vi "AlliGator Color Parameter Map in Original Image.vi"(5 "Color Scale Refnum":refnum<vi>, 7 "Image Color Scale Refnum":refnum<vi>, 8 "Error In":errorcluster, 10 "Destination Image Control Refnum":T1 caption="Source Image Refnum", 11 "AlliGator IV DVR in":refnum<data-value>) -> (0 "Error Out":errorcluster, 1 "# Overlay Pixels":i32, 3 "AlliGator IV DVR out":refnum<data-value>)   [LabVIEW 2021, in "AlliGator Parameter Map.lvlib"]
doc: "Overlays the Decay Fit Parameter Map on the Source Image."
uses:
  AlliGator Parameter Map.lvlib
  Image/Image Control Refnum.ctl
  Internal Variables/AlliGator Internal Variables v2.ctl
  <vilib>/vision/Image Controls.llb/IMAQ Image.ctl
  Internal Variables/AlliGator Gate Image Set.ctl
  Files/AlliGator FLI Dataset Type.ctl
  Files/AlliGator Data Series Type.ctl
  Dual-Channel Datasets/AlliGator Dataset Channel.ctl
  Settings/AlliGator Gate Arithmetic.ctl
  Source Image/AlliGator Displayed Image.ctl
  Image/Named ROI Description.ctl
  Phasor Graph/AlliGator Decay Metadata v3.ctl
  Decay Analysis/Decay Preprocessing/AlliGator Decay Background Subtraction Info.ctl
  Decay Analysis/Decay Preprocessing/AlliGator Baseline Subtraction Method.ctl
  Graphs/XY Graph/XY Graph Plot Shift Parameters.ctl
  Graphs/XY Graph/XY Graph Plot Shift Method.ctl
  Decay Analysis/Decay Preprocessing/AlliGator Decay Extrapolation Parameters.ctl
  Phasor/Calibration Phasor (m, phi).ctl
  Phasor/Phasor Reference Series.ctl
  Phasor/Phasor Calibration Map v2.ctl
  Phasor/Phasor (g, s).ctl
  Phasor Graph/AlliGator Raw Phasor Plot Data v4.ctl
  Phasor/Phasor Standard Deviation Options.ctl
  Phasor Plot/AlliGator Phasor Multi-Harmonic Data.ctl
  Phasor/Phasor Harmonic Data.ctl
  Decay Fit Parameter Map/AlliGator Decay Fit Options & Parameters v2.ctl
  Fits/IRF(X)PSED/Decay Fit Options v2.ctl
  Fits/Decay Convolution/Decay Model.ctl
  Fits/Residual Type.ctl
  Fits/IRF(X)PSED/Fit Weights Type.ctl
  Fits/Non-linear Fitting Method v2.ctl
  Fits/Fit Calculation Method.ctl
  Fits/Non-linear Fitting Algorithm.ctl
  Decay Analysis/Decay Fit/AlliGator Decay Fit Parameter Constraints 2.ctl
  Fits/IRF(X)PSED/Decay Fit Parameters In List.ctl
  Fits/IRF(X)PSED/MLE Baseline Offset Type.ctl
  Decay Analysis/Decay Preprocessing/AlliGator Decay Preprocessing Parameters.ctl
  Fits/IRF(X)PSED/Decay Fit Parameters & Derived Quantities List v2.ctl
  Decay Fit Parameter Map/AlliGator Parameter Maps Data.ctl
  Settings/AlliGator Settings List.ctl
  Globals, Variables, Constants/AlliGator Variables List.ctl
  Palette/Image Palette Information.ctl
  Image/Image Display Palette Type.ctl
  Variant/Variant to Data/Variant to Boolean.vi
  Error/Error.lvlib
  Image/Image.lvlib
  Settings/AlliGator Settings.lvlib
  Variant/Variant to Data/Variant to Data.lvlib
  <vilib>/vision/NI_Vision_Development_Module.lvlib
  Time/Time.lvlib
  Globals, Variables, Constants/AlliGator Globals, Variables & Constants.lvlib
  Palette/Palette.lvlib
  Utilities/Utilities.lvlib
  Phasor/Phasor.lvlib
  Decay Analysis/Decay Preprocessing/AlliGator Decay Preprocessing.lvlib
  Graphs/XY Graph/XY Graph Add-Ons.lvlib
  Phasor Graph/AlliGator Phasor Graph.lvlib
  Files/AlliGator Files.lvlib
  Phasor Plot/AlliGator Phasor Plot.lvlib
  Source Image/AlliGator Source Image.lvlib
  Internal Variables/AlliGator Internal Variables.lvlib
  Fits/Fits.lvlib
  Decay Analysis/Decay Fit/AlliGator Decay Fit.lvlib
  Decay Fit Parameter Map/AlliGator Decay Fit Parameter Map.lvlib
  Dual-Channel Datasets/AlliGator Dual-Channel Datasets.lvlib
panel:
  out "Overlay Copy (s)":dbl
  out "Overlay Erase (s)":dbl
  out "Overlay Compute (s)":dbl
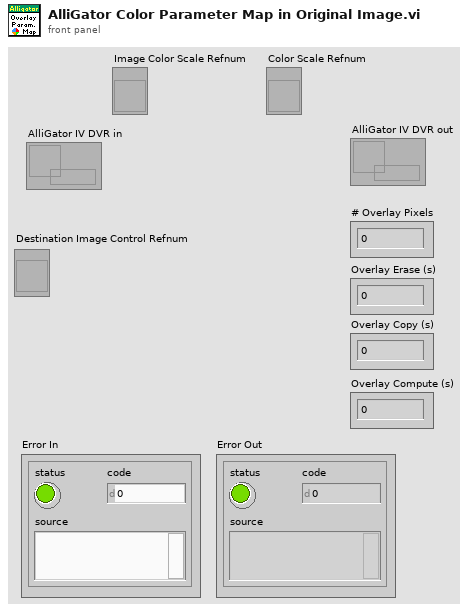
[diagram p1: front panel]
types:
  T1 = typedef "Image.lvlib/Image Control Refnum.ctl" = refnum<vi>
  T2 = typedef "AlliGator Settings.lvlib/AlliGator Settings List.ctl" = enum16{"GUI:Visible Settings Tab", "GUI:Last Run Version", "Source Image:Use Image Histogram for Contrast", "Source Image:Low Count Pixels Rejection Options", "Source Image:High Count Pixels Rejection Options", "Source Image:Use Image Brightness", "Source Image:Blend Overlay with Image Background", "Source Image:Use Fixed ROI Diameter", "Source Image:ROI Diameter", "Source Image:ROI Center Color", "Source Image:Peak Threshold", "Source Image:Intensity Threshold", "Source Image:Image Binning Options", "Source Image:Image Smoothing Options", "Source Image:Image Histogram Active", "Source Image:Invert Binary Mask", "Source Image:Hot Pixel Removal", "Source Image:Overlay Analyzed ROI Center", "Source Image:Auto-Adjust Contrast", "Source Image:Histogram Lower Percentile", "Source Image:Histogram Upper Percentile", "Source Image:Save Source Image", "Source Image:Scale Bar Options", "Source Image:Image Resolution (Pixel Size)", "Source Image:Flatfield Correction", "Source Image:Show Dead Left Columns Correction", "Source Image:Dead Left Columns Correction", "Source Image:Image Pre-Processing Operations Order", "Source Image:Overlay ROI Median", "Source Image:Median Overlay Color", "Data Information:Gate Width", "Data Information:Nanotime Gate Separation", "Data Information:Macrotime Gate Separation", "Data Information:Gate Step", "Data Information:# Gates", "Data Information:Gate Image Exposure", "Data Information:Gate Image Integration", "Data Information:Gates to Skip", "Data Information:Gates to Keep", "Data Information:Define Gates to", "Data Information:Channel Name", "Data Information:Available Channel Names", "Data Information:Channel Arithmetic", "Data Information:Background File Subtraction", "Data Information:Background File", "Data Information:Background Scaling Factor", "Data Information:Background Pile-up Correction", "Data Information:Background Pixel Well Capacity", "Data Information:Laser Period", "Data Information:SYNC Period", "Data Information:Pile-up Correction", "Data Information:Pixel Well Capacity", "Data Information:Dataset Scaling Factor", "Fluorescence Decay_Decay Pre-Processing:Reverse Gates", "Fluorescence Decay_Decay Pre-Processing:Verbose Decay Pre-Processing", "Fluorescence Decay_Decay Pre-Processing:Use Decay Pre-Processing", "Fluorescence Decay_Decay Pre-Processing:Background Subtraction", "Fluorescence Decay_Decay Pre-Processing:Background Definition Range", "Fluorescence Decay_Decay Pre-Processing:Baseline Subtraction Method", "Fluorescence Decay_Decay Pre-Processing:Decay Pre-Processing Operations Order", "Fluorescence Decay_Decay Pre-Processing:Smoothing Parameter", "Fluorescence Decay_Decay Pre-Processing:Shift Decay", "Fluorescence Decay_Decay Pre-Processing:Decay Shift Parameters", "Fluorescence Decay_Decay Pre-Processing:Fold Decay", "Fluorescence Decay_Decay Pre-Processing:# Folds", "Fluorescence Decay_Decay Pre-Processing:1-Normalize Decay", "Fluorescence Decay_Decay Pre-Processing:[0-1]-Normalize Decay", "Fluorescence Decay_Decay Pre-Processing:Smoothen Decay", "Fluorescence Decay_Decay Pre-Processing:Extrapolate Decay", "Fluorescence Decay_Decay Pre-Processing:Use Periodicity", "Fluorescence Decay_Decay Pre-Processing:Use Cursors", "Fluorescence Decay_Decay Pre-Processing:Tail Fraction", "Fluorescence Decay_Decay Pre-Processing:Head Fraction", "Fluorescence Decay_Decay Pre-Processing:Additional Points", "Fluorescence Decay_Decay Pre-Processing:Straighten Decay", "Fluorescence Decay_Decay Pre-Processing:Constant Background", "Fluorescence Decay_Decay Pre-Processing:Pixel-Normalize Decay", "Fluorescence Decay_Advanced Analysis:Extract IRF instead of Decay", "Fluorescence Decay_Advanced Analysis:IRF Extraction Options", "Fluorescence Decay_Advanced Analysis:IRF Optimization Options", "Fluorescence Decay_Advanced Analysis:Square Pulse Options", "Fluorescence Decay_Advanced Analysis:IRF Order", "Fluorescence Decay_Advanced Analysis:IRF Time Constants", "Fluorescence Decay_Advanced Analysis:Wavelet Analysis Options", "Fluorescence Decay_Advanced Analysis:Average Lifetime Options", "Fluorescence Decay_Fit Options:Fit Options", "Fluorescence Decay_Fit Options:Use Legacy Fitting Approach", "Fluorescence Decay_Fit Options:Use Data Information Laser Period", "Fluorescence Decay_Fit Parameters:Displayed Fit Parameters", "Fluorescence Decay_Fit Parameters:Fit Parameter Constraints", "Fluorescence Decay_Fit Parameters:Export Tabulated Results", "Fluorescence Decay_Fit Parameters:MLE Baseline Offset Type", "Fluorescence Decay_Fit Parameters:MLE Baseline Offset", "Fluorescence Decay_Fit Parameters:Guess Parameter Names", "Fluorescence Decay_Fit Parameters:Guess Parameter Values", "Fluorescence Decay_Fit Parameters:Guess Parameters Options", "Fluorescence Decay_Fit Parameters:Optimal Offset Selection Criterion", "Fluorescence Decay_Styles:Show Last Decay Only", "Fluorescence Decay_Styles:Decay Graph Color Array", "Fluorescence Decay:Decay Graph Active", "Fluorescence Decay Statistics:Min Peak Value", "Fluorescence Decay Statistics:Reject Low Decay Peak Pixels", "Fluorescence Decay Statistics:Reject High Decay Peak Pixels", "Fluorescence Decay Statistics:Max Peak Value", "Time Traces:Use File Timestamp", "Time Traces:Time Step", "Time Traces:Use Intensity Correction File", "Time Traces:Intensity Correction File", "Phasor Plot:Phasor Plot Smoothing Options", "Phasor Plot:Phasor Plot Size", "Phasor Plot:Phasor Plot Graphics Options", "Phasor Plot:Cumulative Phasor Plot", "Phasor Plot:Use Phasor Brightness", "Phasor Plot:Blend Overlay with Phasor Background", "Phasor Plot:Save Phasor Plot", "Phasor Plot:Show References", "Phasor Plot:Phasor Ratio Decay Range", "Phasor Plot:Exponential Fading", "Phasor Plot:Phasor Ratio Reference Colors", "Phasor Plot:Reference Radius", "Phasor Plot:Show Color Map Vertices", "Phasor Plot:Phasor Plot Active", "Phasor Plot:Phasor Ratio Color Map Type", "Phasor Plot:Phasor Ratio Color Map", "Phasor Plot:Phasor Ratio Display Range", "Phasor Plot:Selected Image ROI(s)", "Phasor Plot:All Image ROIs", "Phasor Plot:Selected Phasor Plot ROI(s)", "Phasor Plot:All Phasor Plot ROIs", "Phasor Plot:Phasor Ratio Color-Coded Quantity", "Phasor Plot:Store Phasor Harmonics", "Phasor Plot:Draw Reference Segment", "Phasor Plot:User-Defined Quantity", "Phasor Plot:Color Scale High Color", "Phasor Plot:Color Scale Low Color", "Phasor Graph:Phasor Frequency", "Phasor Graph:Phasor Ratio Type", "Phasor Graph:Pixel-level Phasor Computation", "Phasor Graph:Save Phasor Graph", "Phasor Graph:Phasor Graph Active", "Phasor Graph:Phasor SDV Options", "Phasor Calibration:Use Backup Calibration if needed", "Phasor Graph:Define Shortest Lifetime as", "Phasor Calibration:Backup Calibration Type", "Phasor Calibration:Calibration Type", "Phasor Calibration:Calibration Lifetime", "Phasor Calibration:Calibration Map Algorithm", "Single-Exponential Phasor Locus (SEPL):Gate Parameters", "Single-Exponential Phasor Locus (SEPL):User-defined Gate", "Single-Exponential Phasor Locus (SEPL):User-defined IRF", "Single-Exponential Phasor Locus (SEPL):Phasor Parameters", "Single-Exponential Phasor Locus (SEPL):Decay & IRF Parameters", "Single-Exponential Phasor Locus (SEPL):Display Parameters", "Lifetime Analysis:Decay Analysis Parameters", "Lifetime Analysis:Lifetime Map Active", "Plugins:Python Settings", "Miscellaneous:Verbose Mode", "Miscellaneous:Beep after Script", "Miscellaneous:Saved Image File Format", "Miscellaneous:Exported Gate Image Settings", "Miscellaneous:Include Loading in Timing", "Miscellaneous:Verbose Settings Mode", "Miscellaneous:Histogram Options", "Miscellaneous:Beep on Error", "Miscellaneous:# Logical Processors Used", "Miscellaneous:ROI Description Max Characters", "Miscellaneous:Verbose Error Mode", "Miscellaneous:Transparent Mask Color"}
  T3 = typedef "IMAQ Image.ctl" = refnum<image>
  T4 = typedef "AlliGator Globals, Variables & Constants.lvlib/AlliGator Variables List.ctl" = enum16{"---- GUI ----", "GUI:Initialization Status", "GUI:State Indicators Refnum", "GUI:Original AlliGator Menu Items", "GUI:Current Action Loop State", "GUI:Script in progress", "GUI:Playback", "GUI:Loop Playback", "GUI:Search ROI Used", "GUI:Search ROI", "Decay Graph Max Legend Size", "Intensity Graph Max Legend Size", "Decay Statistics Graph Max Legend Size", "Phasor Graph Max Legend Size", "Phasor Ratio Graph Max Legend Size", "Lifetime Graph Max Legend Size", "---- Files ----", "Files:Export Dataset Frames as Individual Files", "Files:Show Batch Export Help Balloons", "Files:Frames in Dataset", "Files:ptu File Frame Start Indices", "Files:Current Frame in Dataset", "Files:Current Frame Timestamp", "Files:Dataset Loaded", "Files:Dataset Metadata", "Files:Dataset Channel", "Files:Dataset Data Description", "Files:Background Dataset Metadata", "Files:Background Dataset Channel", "Files:Background Dataset Data Description", "Files:Background File Subtraction", "Files:Background File Path", "Files:Background File Pile-up Correction", "Files:Background File Pixel Well Capacity", "Files:Background File Scaling Factor", "Files:Current Dataset Load Settings", "Files:Dataset Path", "Files:ICCD-specific Information", "Files:Macrotime Gate Separation", "------ Python Plugins ------", "Python Plugins:Information", "Python Plugins:Python Session", "Python Plugins:Valid Python Session?", "---- Source Image ----", "Source Image:ROIs", "Source Image:Current ROI", "Source Image:ROI Event Refnum", "X_Source Image:Display Range", "X_Source Image:Palette Information", "X_Source Image:Type of Displayed Image", "X_Time Gate Slider", "Source Image:Palette List", "Source Image:Scale", "Source Image:ROI Overlay Color", "Source Image:Overlay to Erase", "Source Image:Is Displayed Image Accumulated", "Source Image:White Light Image Modified", "Source Image:Mask Image Modified", "---- Image Profile Window ----", "Image Profile:Window Event Refnum", "Image Profile:IntensityType", "Image Profile:Intensity Average Type", "Image Profile:Intensity-weighted SDV", "Image Profile:Box Profile Type", "Image Profile:Window Open", "Image Profile:Plotted Fit Parameter", "------ Phasor Graph -------", "Phasor Graph:Show Line", "---- Phasor Plot ---", "Phasor Plot:Parameters Changed", "Phasor Plot:FLI Dataset Modified since last Calculation", "Phasor Harmonics Data", "Selected Phasor Harmonics", "Phasor Harmonic Manager Event Refnum", "Phasor Plot:ROIs", "Phasor Plot:Current ROI", "Phasor Plot:ROI Event Refnum", "Phasor Plot:Image Reference Points", "Phasor Plot:Computed", "Phasor Plot:Palette Information", "Phasor Plot:Palette List", "Phasor Plot:Phasor Ratio Palette Information", "Phasor Plot:Phasor Ratio Palette List", "Phasor Plot:Image Scale", "Phasor Plot:Image Overlay to Erase", "Phasor Plot:Image Elements to Update", "Phasor Plot:Current Calculation Parameters", "Phasor Plot:Current Calibration Options", "Phasor Plot:Reset Cumulated Phasor Plot", "Phasor Plot:Reference 1", "Phasor Plot:Lifetime Reference 1", "Phasor Plot:Reference 1 Frequency", "Phasor Plot:Reference 2", "Phasor Plot:Lifetime Reference 2", "Phasor Plot:Reference 2 Frequency", "---- Decay Analysis ----", "Number of Selected Decays to Fit", "LS Fit Results", "LAR Fit Results", "BS Fit Results", "Last Decay Max - Min", "Best Fit Parameters", "Best Fit Parameter Names", "Actual Size X", "Actual Size Y", "Binning X", "Binning Y", "Actual # Gates", "Dataset Number", "Gates to...", "Gates Skipped", "Gates to keep", "Gate Step", "Gate Separation", "Reversed Gates", "Pile-up Correction", "Pixel Well Capacity", "Background Subtracted", "Background Subtraction Method", "Background Definition Range", "Background File (deprecated)", "Number of Dataset Accumulated", "Array of Accumulated Dataset Paths", "Do Averaged Datasets", "Destination File Path", "Process Plot Target", "Use 1/D as Phasor Frequency", "---- Decay Fit Parameter Map -----", "Decay Fit Parameter Map:Palette Information", "Decay Fit Parameter Map:Palette List", "Decay Fit Parameter Map:X Resolution", "Decay Fit Parameter Map:Y Resolution", "---- Parameter Map ----", "Parameter Map:Palette Information", "Parameter Map:Palette List", "------- Local Decay Window ---------", "Local Decay Graph Window:Event Refnum", "Local Decay Graph Window:Use normalized IRF for convolution", "----- Miscellaneous ----", "Misc:Skippable Dialog Windows Status"}
  T5 = typedef "Palette.lvlib/Image Palette Information.ctl" = cluster{"Palette Name [# Colors,int?,inv?]":string, "Palette Type":T6, "Palette Colors":u32[], "Interpolate?":bool}
  T6 = typedef "Image.lvlib/Image Display Palette Type.ctl" = u32
  T7 = typedef "AlliGator Internal Variables.lvlib/AlliGator Internal Variables v2.ctl" = cluster{"Displayed Image":T3, "White Light Image":T3, "Mask Image":T3, "ROI Mask Image":T3, "Current Dataset Images 1":T8, "Background Dataset Images 1":T8, "Current Dataset Images 2":T8, "Background Dataset Images 2":T8, "Current Dataset Arithmetic Images":T8, "Accumulated Dataset Images 1":T8, "Accumulated Dataset Images 2":T8, "Accumulated Dataset Arithmetic Images":T8, "Phasor Plot Image":T3, "Decay Fit Parameter Map Image":T3, "Parameter Map Image":T3, "Single Data Point Path":path, "White Light Image Path":path, "Mask Image Path":path, "Time-Series Folder":path, "[Time-Series Paths]":path[], "Current Dataset":i32, "Single Dataset Type":T9, "Current Folder":string, "AlliGator Data Series Type":T10, "# Datasets":i32, "Dual-Channel Dataset":bool, "Selected Channel Name":string, "Dataset Channel":T11, "Channel Arithmetic":T12, "Dual-Channel Background Dataset":bool, "Background Channel":T11, "Dual-Channel Accumulated Dataset":bool, "Start Time":dbl, "[Time-Series Timestamps]":dbl[], "[Intensity Corrections]":dbl[], "Time Series Script":bool, "Type of Displayed Image":T13, "Gate Image Slide":u16, "# Gates":i32, "ROIs":T14[], "ROI Decay":cluster{"t Array":dbl[], "I Array":dbl[]}, "Valid Decay":bool, "Decay  Metadata":T16, "Reference Decay Plot Name":string, "Reference Decay":cluster{"t Array":dbl[], "I Array":dbl[]}, "Decay Shift Plot":cluster{"Time Stamps":dbl[], "Decay Shifts":dbl[]}, "[Decays Max Values]":sgl[], "[Decays Min Values]":sgl[], "Calibration Phasor":T22, "Calibration Phasor Series":T23, "Phasor Calibration Map":T24, "Calibration Map MD5 Digest":string, "Last Raw Phasor":T25, "Last Calibrated Phasor":T25, "Last Calibrated Phasor SDV":T25, "Phasor Graph:Phasor Plot":cluster{"g Array":dbl[], "s Array":dbl[]}, "Phasor Graph:Phasor SDV Plot":cluster{"g Array":dbl[], "s Array":dbl[]}, "[Phasor Graph:Raw Phasor Plots]":T26[], "Phasor Plot locked to Ref 1":i32, "[Phasor Plot(s) locked to Ref 1]":i32[], "[Phasor Plot(s) locked to Ref 2]":i32[], "[Pixel Phasors]":T25[], "[[Sum Image]]":dbl[][], "[[CSG Phasors]]":csg[][], "[[Valid Pixel?]]":bool[][], "I/m/phi Dataset":cluster{"I/m/phi Dataset?":bool, "Base Frequency":dbl[unit], "Harmonic Orders":u8[]}, "Multi Phasor Plot Data":T28, "Decay Fit Options & Parameters":T30, "Fit Options: Decay Preprocessing Parameters":T41, "Fit Options: Reference Decay":cluster{"t Array":dbl[], "I Array":dbl[]}, "Is Full Image Parameters Map":bool, "Is Single-Pixels Parameters Map":bool, "NLSF Parameters Map X Resolution":i32, "NLSF Parameters Map Y Resolution":i32, "[Single Decay Fit Parameters]":dbl[], "Fit Model":T32, "[[Multiple Decays Fit Parameters]]":dbl[][], "[[Multiple Decays Fit Parameter SDVs]]":dbl[][], "[[IRFs]]":dbl[][], "IRF Array Time Axis":dbl[], "Decay Array Time Axis":dbl[], "[Decay Fit Parameter Names]":T42[], "[[Phasor Ratios]]":dbl[][], "[[Average Lifetimes]]":dbl[][], "Amplitude Weighted Average Lifetime":bool, "[Decay Sum]":dbl[], "[Map Set Names]":string[], "[Parameter Maps]":T43[], "[[User-defined Quantities]]":dbl[][], "User-defined Quantity":string}
  T8 = typedef "AlliGator Internal Variables.lvlib/AlliGator Gate Image Set.ctl" = cluster{"SGL Image Max":T3, "SGL Image Sum":T3, "SGL Gate Images":T3[], "SGL Image Min":T3}
  T9 = typedef "AlliGator Files.lvlib/AlliGator FLI Dataset Type.ctl" = enum16{"HDF5 FLI Dataset", "Gate Image Folder", ".sdt FLI Dataset (Becker & Hickl)", ".ptu FLI Dataset (PicoQuant)", "SS1 FLI Dataset", "SS2 FLI Dataset", "I/m/phi Dataset", ".bin FLI Dataset (PicoQuant Binned)", ".bin FLI Dataset (Piccolo Binned)", ".mat FLI Dataset"}
  T10 = typedef "AlliGator Files.lvlib/AlliGator Data Series Type.ctl" = enum16{"Not a Supported Series", "Gate Images Folder Series", "SwissSPAD 2 Dataset Series", "B&H FLI Dataset Series", "PicoQuant PTU FLI Dataset Series", "PicoQuant BIN FLI Dataset Series", "Piccolo hist BIN FLI Dataset Series", "HDF5 FLI Dataset Series"}
  T11 = typedef "AlliGator Dual-Channel Datasets.lvlib/AlliGator Dataset Channel.ctl" = enum16{"G2", "INT"}
  T12 = typedef "AlliGator Settings.lvlib/AlliGator Gate Arithmetic.ctl" = enum16{"None", "INT-G2", "G2/INT*<INT>", "(1 - G2/INT)*<INT>"}
  T13 = typedef "AlliGator Source Image.lvlib/AlliGator Displayed Image.ctl" = enum16{"Single Gate", "Sum of All Gates", "Max of All Gates", "Min of All Gates", "-", "White Ligth Image", "Mask Image"}
  T14 = typedef "Image.lvlib/Named ROI Description.ctl" = cluster{"ROI Descriptor":T15, "ROI Name":string, "Overlay Color":u32}
  T15 = typedef "ROI Descriptor" = cluster{"Global Rectangle":i32[], "Contours":cluster{"ID":enum32{"External", "Internal"}, "Type":u32, "Coordinates":i32[]}[]}
  T16 = typedef "AlliGator Phasor Graph.lvlib/AlliGator Decay Metadata v3.ctl" = cluster{"ROI Descriptor":T15, "ROI Center":cluster{"X":i32, "Y":i32}, "Decay Background Subtraction Info":T17, "Decay Reverted":bool, "Decay Smoothened":bool, "Decay Straightened":bool, "Fitted Tau (Decay Straightening)":dbl, "Decay Shift Parameters":T19, "Decay Shifted":bool, "Decay Extrapolated":bool, "Decay Extrapolation Parameters":T21, "Decay Normalized":bool, "Fold Decay":bool, "# Folds":u32}
  T17 = typedef "AlliGator Decay Preprocessing.lvlib/AlliGator Decay Background Subtraction Info.ctl" = cluster{"Laser Period":dbl[unit], "Gate Duration":dbl[unit], "Baseline Subtraction Method":T18, "Background Definition Range":cluster{"Min Gate":dbl[unit], "Max Gate":dbl[unit]}, "Total Intensity w/o Bkgd Subtraction":dbl, "Bkgd-subtracted Intensity (exp)":dbl, "# Data Points":i32, "Background/Gate":dbl, "Fitted Lifetime":dbl[unit], "Bkgd-subtracted Intensity (theo)":dbl}
  T18 = typedef "AlliGator Decay Preprocessing.lvlib/AlliGator Baseline Subtraction Method.ctl" = enum16{"Mean", "Min", "Square Gated Single-Exponential", "File", "Constant"}
  T19 = typedef "XY Graph Add-Ons.lvlib/XY Graph Plot Shift Parameters.ctl" = cluster{"Type":T20, "Shift":dbl[unit], "Threshold":dbl, "Rotate":bool}
  T20 = typedef "XY Graph Add-Ons.lvlib/XY Graph Plot Shift Method.ctl" = enum16{"Default", "CFD", "Threshold", "Cross-Correlation"}
  T21 = typedef "AlliGator Decay Preprocessing.lvlib/AlliGator Decay Extrapolation Parameters.ctl" = cluster{"Additional Points":u32, "Head Fraction":dbl, "Fitted Tau":dbl, "Use Periodicity":bool, "Use Cursors":bool, "Tail Fraction":dbl}
  T22 = typedef "Phasor.lvlib/Calibration Phasor (m, phi).ctl" = cluster{"m":dbl, "phi":dbl, "Phasor Frequency":dbl[unit], "Reference Lifetime":dbl[unit]}
  T23 = typedef "Phasor.lvlib/Phasor Reference Series.ctl" = cluster{"m Array":dbl[], "phi Array":dbl[], "Phasor Frequency":dbl[unit], "Calibration Lifetime":dbl[unit]}
  T24 = typedef "Phasor.lvlib/Phasor Calibration Map v2.ctl" = cluster{"Phasor Frequency":dbl[unit], "Calibration Lifetime":dbl[unit], "ROI Centers":cluster{"X":i32, "Y":i32}[], "ROI Descriptors":T15[], "Map Resolution X":i32, "Map Resolution Y":i32, "z Array":cdb[]}
  T25 = typedef "Phasor.lvlib/Phasor (g, s).ctl" = cluster{"g":dbl, "s":dbl}
  T26 = typedef "AlliGator Phasor Graph.lvlib/AlliGator Raw Phasor Plot Data v4.ctl" = cluster{"Phasor Plot Name":string, "Raw Phasor Plot":T25[], "Phasor Frequency":dbl[unit], "[Decay Metadata]":T16[], "Raw Phasor Plot SDV":T25[], "Phasor SDV Options":T27, "[Calibration Phasor]":T22[]}
  T27 = typedef "Phasor.lvlib/Phasor Standard Deviation Options.ctl" = cluster{"Compute Estimated SDV":bool, "# Replicas":u32, "Use Estimated Average Phasor":bool}
  T28 = typedef "AlliGator Phasor Plot.lvlib/AlliGator Phasor Multi-Harmonic Data.ctl" = cluster{"Base Frequency":dbl[unit], "# Harmonics":u8, "Harmonic Orders":u8[], "Phasor Plot Settings Checksum":u64, "Phasor Harmonic Data Array":T29[]}
  T29 = typedef "Phasor.lvlib/Phasor Harmonic Data.ctl" = cluster{"Phasor Harmonic Name":string, "Phasor Plot Settings Checksum":u64, "Phasor Frequency":dbl[unit], "Base Frequency":dbl[unit], "Harmonic Order":u8, "Phasor Plot Parameters":string, "Phasor Array [[CSG]]":csg[][], "Dataset File Path":path}
  T30 = typedef "AlliGator Decay Fit Parameter Map.lvlib/AlliGator Decay Fit Options & Parameters v2.ctl" = cluster{"SYNC Period":dbl[unit], "Fit Options":T31, "Fit Parameter Constraints":T38[], "MLE Baseline Offset":dbl, "MLE Baseline Offset Type":T40}
  T31 = typedef "Fits.lvlib/Decay Fit Options v2.ctl" = cluster{"Show Fit Residuals":bool, "Fit Model":T32, "Residual Type":T33, "Max Decay Percentile":dbl, "Min Decay Percentile":dbl, "Show Full Decay":bool, "Weights":T34, "Fitting Method":T35, "Compute Parameter Uncertainties":bool, "Periodic Boundaries":bool, "Model Calculation":T36, "Period":dbl[unit], "Termination Criteria":cluster{"Max Iterations":i32, "Max Function Calls":i32, "Max Time":dbl[unit], "Function Tolerance":dbl, "Parameter Tolerance":dbl, "Gradient Tolerance":dbl, "Min Lambda":dbl, "Max Lambda":dbl, "Initial Tick Count":u32}, "Offset Resolution":dbl[unit], "Use Local IRF":bool, "Fitting Algorithm":T37}
  T32 = typedef "Fits.lvlib/Decay Model.ctl" = enum16{"1-Exponential", "2-Exponentials"}
  T33 = typedef "Fits.lvlib/Residual Type.ctl" = enum16{"Standard", "Normalized", "Reduced"}
  T34 = typedef "Fits.lvlib/Fit Weights Type.ctl" = enum16{"Unweighted", "1/Variance", "Best of All"}
  T35 = typedef "Fits.lvlib/Non-linear Fitting Method v2.ctl" = enum16{"Least Square", "Least Absolute Residual", "Bisquare", "MLE", "-", "Best of All"}
  T36 = typedef "Fits.lvlib/Fit Calculation Method.ctl" = enum16{"Simulation", "Convolution", "Integration"}
  T37 = typedef "Fits.lvlib/Non-linear Fitting Algorithm.ctl" = enum16{"Levenberg-Marquardt", "Trust-Region Dogleg"}
  T38 = typedef "AlliGator Decay Fit.lvlib/AlliGator Decay Fit Parameter Constraints 2.ctl" = cluster{"Fit Parameter":T39, "Min Value":dbl, "Max Value":dbl, "Global":bool, "Used":bool}
  T39 = typedef "Fits.lvlib/Decay Fit Parameters In List.ctl" = enum16{"Offset", "Baseline", "A_1", "tau_1", "A_2", "tau_2"}
  T40 = typedef "Fits.lvlib/MLE Baseline Offset Type.ctl" = enum32{"Absolute", "Percentage"}
  T41 = typedef "AlliGator Decay Preprocessing.lvlib/AlliGator Decay Preprocessing Parameters.ctl" = cluster{"Background Subtraction":bool, "Straighten Decay":bool, "Reverse Gates":bool, "1-Normalized Decay":bool, "Smoothen Decay":bool, "Smoothing Parameter":dbl, "Shift Decay":bool, "Decay Shift Parameters":T19, "Extrapolate Decay":bool, "Additional Points":u32, "Head Fraction":dbl, "Pixel-Normalize Decay":bool, "Use Periodicity":bool, "Use Cursors":bool, "Tail Fraction":dbl, "Use Decay Pre-Processing":bool, "Fold Decay":bool, "# Folds":u32, "[0-1]-Normalized Decay":bool}
  T42 = typedef "Fits.lvlib/Decay Fit Parameters & Derived Quantities List v2.ctl" = enum16{"Offset", "Baseline", "A_1", "tau_1", "A_2", "tau_2", "<tau>_a", "f1_a", "f2_a", "<tau>_i", "f1_i", "f2_i", "-", "R^2", "Chi^2"}
  T43 = typedef "AlliGator Decay Fit Parameter Map.lvlib/AlliGator Parameter Maps Data.ctl" = cluster{"Map Set Name":string, "[Parameter Names]":string[], "[[Parameters]]":dbl[][], "[[Parameter SDVs]]":dbl[][], "Decay Array Time Axis":dbl[], "[[IRFs]]":dbl[][], "IRF Array Time Axis":dbl[]}
  T44 = cluster{"Red (or Hue) value":u8, "Green (or Sat) value":u8, "Blue (or Light or Val) value":u8}[]
  T45 = cluster{"Red (or Hue) value":u8, "Green (or Sat) value":u8, "Blue (or Light or Val) value":u8}
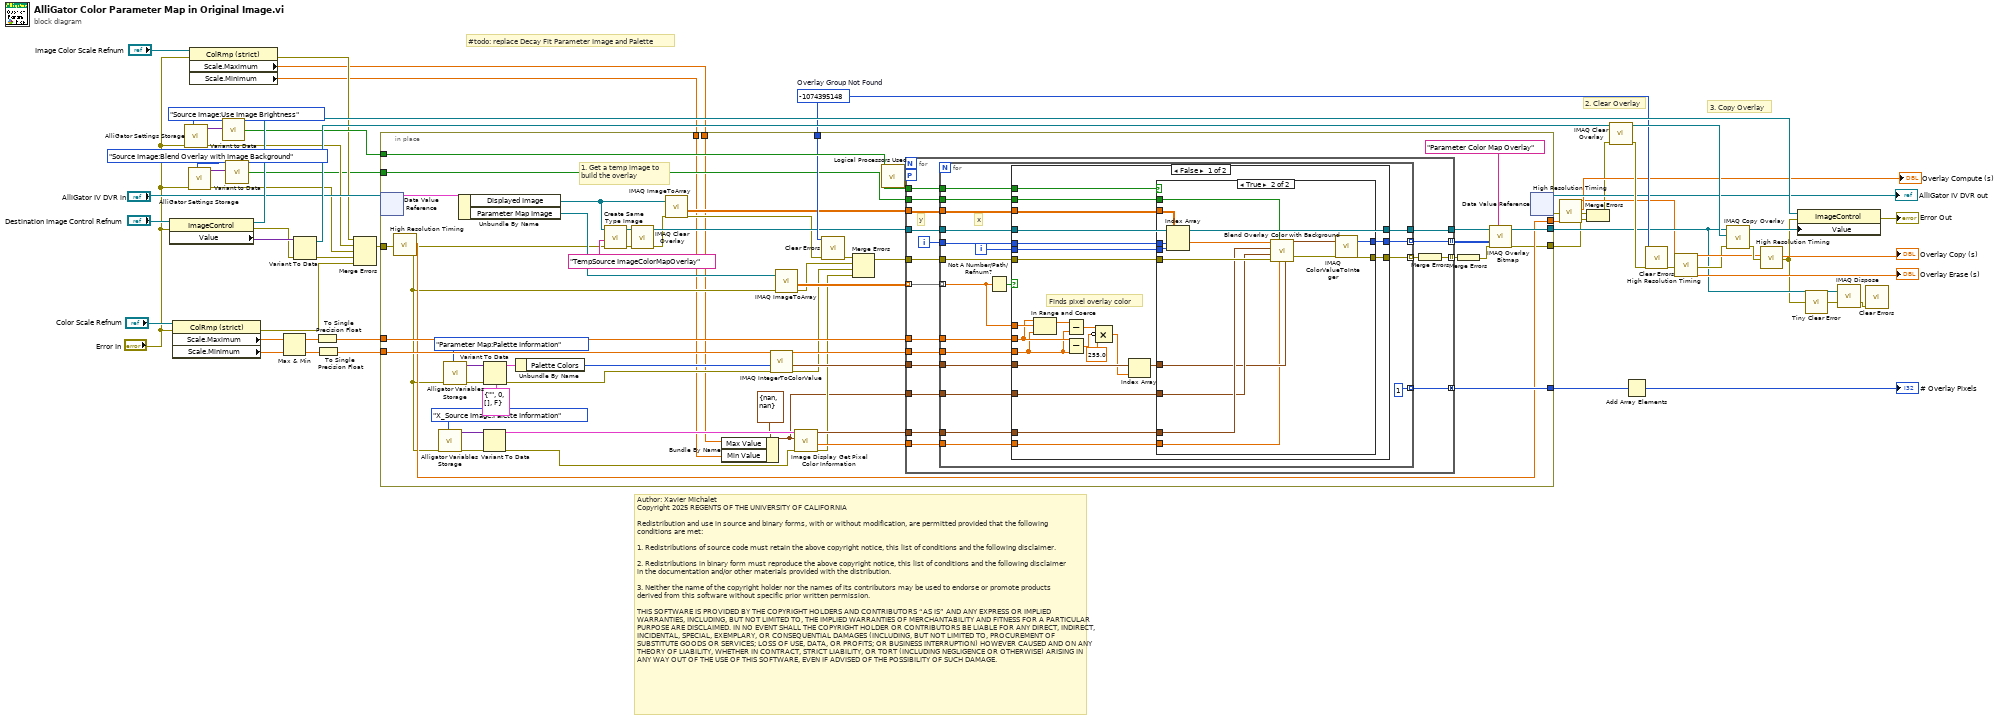
[diagram p0: block diagram]
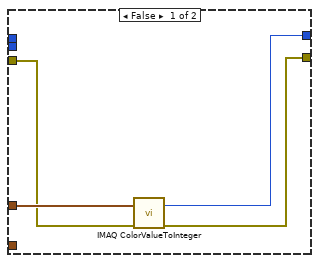
[diagram p2: hidden frame]
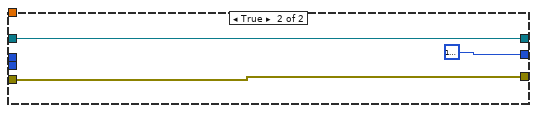
[diagram p3: hidden frame]
diagram:
  w40 = -1074395148  # Overlay Group Not Found
  # "#todo: replace Decay Fit Parameter Image and Palette"
  # "Author: Xavier Michalet\nCopyright 2025 REGENTS OF THE UNIVERSITY OF CALIFORNIA\n\nRedistribution and use in source and binary forms, with or without modification, are permitted provided that the following conditions are met:\n\n1. Redistributions of source code must retain the above copyright notice, this list of conditions and the following disclaimer.\n\n2. Redistributions in binary form must reproduce the above copyright notice, this list of conditions and the following disclaimer in the documentation and/or other materials provided with the distribution.\n\n3. Neither the name of the copyright holder nor the names of its contributors may be used to endorse or promote products derived from this software without specific prior written permission.\n\nTHIS SOFTWARE IS PROVIDED BY THE COPYRIGHT HOLDERS AND CONTRIBUTORS “AS IS” AND ANY EXPRESS OR IMPLIED WARRANTIES, INCLUDING, BUT NOT LIMITED TO, THE IMPLIED WARRANTIES OF MERCHANTABILITY AND FITNESS FOR A PARTICULAR PURPOSE ARE DISCLAIMED. IN NO EVENT SHALL THE COPYRIGHT HOLDER OR CONTRIBUTORS BE LIABLE FOR ANY DIRECT, INDIRECT, INCIDENTAL, SPECIAL, EXEMPLARY, OR CONSEQUENTIAL DAMAGES (INCLUDING, BUT NOT LIMITED TO, PROCUREMENT OF SUBSTITUTE GOODS OR SERVICES; LOSS OF USE, DATA, OR PROFITS; OR BUSINESS INTERRUPTION) HOWEVER CAUSED AND ON ANY THEORY OF LIABILITY, WHETHER IN CONTRACT, STRICT LIABILITY, OR TORT (INCLUDING NEGLIGENCE OR OTHERWISE) ARISING IN ANY WAY OUT OF THE USE OF THIS SOFTWARE, EVEN IF ADVISED OF THE POSSIBILITY OF SUCH DAMAGE."
  # "3. Copy Overlay"
  # "2. Clear Overlay"
  n1 = property class="ImageControl"(reference="Destination Image Control Refnum", error in="Error In") -> (reference out=w50:T1, error out=w52:errorcluster, "Value"=w53:variant)
  n2 = property class="ColRmp (strict)"(reference="Color Scale Refnum", error in="Error In") -> (error out=w22:errorcluster, "Scale.Maximum"=w20:dbl, "Scale.Minimum"=w19:dbl)  [unwired: 1 out]
  n3 = call "AlliGator Settings Storage.vi"("AlliGator Settings List"=AlliGator_Settings_List."Source Image:Use Image Brightness", "Error In"="Error In") -> ("Error Out"=w25:errorcluster, "Variant Data out"=w45:variant)  [unwired: 8 in]
  n4 = call "AlliGator Settings Storage.vi"("AlliGator Settings List"=AlliGator_Settings_List."Source Image:Blend Overlay with Image Background", "Error In"="Error In") -> ("Error Out"=w10:errorcluster, "Variant Data out"=w13:variant)  [unwired: 8 in]
  n5 = property class="ColRmp (strict)"(reference="Image Color Scale Refnum", error in="Error In") -> (error out=w24:errorcluster, "Scale.Maximum"=w2:dbl, "Scale.Minimum"=w1:dbl)  [unwired: 1 out]
  n6 = call-poly "Variant to Data.vi"("Variant"=w45) -> ("Value"=w42:bool)  [unwired: 8 in]
  n7 = call-poly "Variant to Data.vi"("Variant"=w13) -> ("Value"=w9:bool)  [unwired: 8 in]
  n8 = Max & Min(x=w20, y=w19) -> (max(x,y)=w18:dbl, min(x,y)=w17:dbl)
  n9 = Variant To Data(error in=w52, Variant=w53) -> (data=w44:T3, error out=w43:errorcluster)  [unwired: 1 in]
  n10 = To Single Precision Float(number=w18) -> (single precision float=w16:sgl)
  n11 = To Single Precision Float(number=w17) -> (single precision float=w15:sgl)
  n12 = Merge Errors(w24, w25, w10, w43, w22) -> (w26:errorcluster)
  n13 = in-place {
    in-place-border: [w106] -> w49
    in-place-border: [w105] -> w30
    in-place-border: w26 -> [w104]
    in-place-border: w42 -> [w103]
    in-place-border: w40 -> [w102]
    in-place-border: w16 -> [w100]
    in-place-border: w15 -> [w99]
    in-place-border: w9 -> [w80]
    in-place-border: [w79] -> w7
    in-place-border: [w63] -> w3
    in-place-border: w2 -> [w57]
    in-place-border: w1 -> [w56]
    # "1. Get a temp image to\nbuild the overlay"
    n14 = in-place-dvr #1("AlliGator IV DVR in") -> (w101:T7)  [unwired: 1 out]
    n15 = call "High Resolution Timing.vi"("Error In"=w104) -> ("elapsed (relative) seconds"=w79:dbl, "Error Out"=w73:errorcluster)  [unwired: 16 in, 1 out]
    n16 = call "Alligator Variables Storage.vi"("AlliGator Variable"=AlliGator_Variables_List."X_Source Image:Palette Information" ("Alligator Variable"), "Error In"=w73) -> ("Error Out"=w76:errorcluster, "Data out"=w77:variant)  [unwired: 7 in, 1 out]
    n17 = call "Alligator Variables Storage.vi"("AlliGator Variable"=AlliGator_Variables_List."Parameter Map:Palette Information" ("Alligator Variable"), "Error In"=w73) -> ("Error Out"=w90:errorcluster, "Data out"=w91:variant)  [unwired: 7 in, 1 out]
    n18 = Unbundle By Name(w101) -> ("Displayed Image"=w81:T3, "Parameter Map Image"=w85:T3)
    n19 = Variant To Data(error in=w76, Variant=w77) -> (data=w78:T5, error out=w70:errorcluster)  [unwired: 1 in]
    n20 = Variant To Data(error in=w90, type=T5 {"Palette Name [# Colors,int?,inv?]"="", "Palette Type"=0, "Palette Colors"=[], "Interpolate?"=FALSE} ("Image Display Palette Information"), Variant=w91) -> (data=w88:T5, error out=w69:errorcluster)
    n21 = Unbundle By Name(w88) -> ("Palette Colors"=w87:u32[])
    n22 = call "Create Same Type Image.vi"("error in (no error)"=w73, "Name in"="TempSource ImageColorMapOverlay", "Image Src"=w81) -> ("error out"=w95:errorcluster, "Image Dst"=w97:T3)  [unwired: 6 in, 1 out]
    n23 = call "IMAQ Clear Overlay"("error in (no error)"=w95, "Image"=w97) -> ("error out"=w83:errorcluster, "Image Out"=w96:T3)  [unwired: 8 in]
    n24 = call "IMAQ ImageToArray"("error in (no error)"=w83, "Image"=w81) -> ("Image Pixels (Float)"=w64:sgl[][], "error out"=w82:errorcluster)  [unwired: 2 in, 3 out]
    n25 = Bundle By Name(cluster=cluster{"Min Value":sgl, "Max Value":sgl} {"Min Value"=nan, "Max Value"=nan} ("Image Display Range"), "Max Value"=w57, "Min Value"=w56) -> (w55:cluster{"Min Value":sgl, "Max Value":sgl})
    n26 = call "IMAQ IntegerToColorValue"("error in (no error)"=w69, "1D U32 array"=w87) -> ("1D Color value array"=w86:T44, "error out"=w66:errorcluster)  [unwired: 3 in, 2 out]
    n27 = call "IMAQ ImageToArray"("error in (no error)"=w73, "Image"=w85) -> ("Image Pixels (Float)"=w84:sgl[][], "error out"=w67:errorcluster)  [unwired: 2 in, 3 out]
    n28 = call "Image Display Get Pixel Color Information.vi"("Error In"=w70, "Image Display Range"=w55, "Image Display Palette Information"=w78) -> ("Error Out"=w65:errorcluster, "Image Scale Factor (256 colors)"=w71:sgl, "1D Color Array"=w72:cluster{"Red":u8, "Green":u8, "Blue":u8}[])  [unwired: 5 in, 1 out]
    n29 = call <vilib>:"Clear Errors.vi"("error in (no error)"=w82, "specific error code to clear (0: all)"=w102) -> ("error out"=w94:errorcluster)  [unwired: 4 in, 1 out]
    n30 = Merge Errors(w94, w67, w66, w65) -> (w68:errorcluster)
    n31 = call "Logical Processors Used.vi"() -> ("# Logical Processor Used"=w62:i32)  [unwired: 6 in]
    n32 = for {
      tunnel: w103 -> [w119]
      tunnel: w68 -> [w122]
      tunnel: [w120] -> w106 mode=concatenating
      tunnel: w100 -> [w118]
      tunnel: w99 -> [w117]
      tunnel: w86 -> [w116]
      tunnel: w96 -> [w123]
      tunnel: [w121] -> w61
      tunnel: w84 -> [w115] mode=indexing
      tunnel: w64 -> [w114]
      workers-P: w62 -> [_]
      tunnel: w80 -> [w113]
      tunnel: w72 -> [w112]
      tunnel: w71 -> [w111]
      tunnel: [w110] -> w59 mode=indexing
      tunnel: [w108] -> w60 mode=indexing
      tunnel: w55 -> [w107]
      i -> [w124]
      # "y"
      n33 = for {
        tunnel: w124 -> [w138]
        tunnel: w119 -> [w139]
        tunnel: w122 -> [w142]
        tunnel: [1] -> w120 mode=indexing
        tunnel: w118 -> [w136]
        tunnel: w117 -> [w135]
        tunnel: w116 -> [w134]
        tunnel: w123 -> [w143]
        tunnel: [w141] -> w121
        tunnel: w115 -> [w131] mode=indexing
        tunnel: w114 -> [w132]
        tunnel: w113 -> [w130]
        tunnel: w112 -> [w129]
        tunnel: w111 -> [w128]
        tunnel: [w127] -> w110 mode=indexing
        tunnel: [w126] -> w109 mode=indexing
        tunnel: w107 -> [w125]
        i -> [w137]
        # "x"
        n34 = Not A Number/Path/Refnum?(number/path/refnum=w131) -> (NaN/Path/Refnum?=w133:bool)
        n35 = case shown="False" w133 {
          tunnel: w143 -> [w147 w186]
          tunnel: [w145 w185] -> w126
          tunnel: [w147 w186] -> w141
          tunnel: w139 -> [w165 _]
          tunnel: w138 -> [w164 _]
          tunnel: w137 -> [w163 _]
          tunnel: w142 -> [w162 w185]
          tunnel: w136 -> [w160 _]
          tunnel: w135 -> [w158 _]
          tunnel: w131 -> [w161 _]
          tunnel: w134 -> [w154 _]
          tunnel: w132 -> [w151 _]
          tunnel: w130 -> [w150 _]
          tunnel: w129 -> [w149 _]
          tunnel: w128 -> [w148 _]
          tunnel: [w146 u32 16777216] -> w127
          tunnel: w125 -> [w144 _]
          frame False {
            # "Finds pixel overlay color"
            n36 = In Range and Coerce(upper limit=w160, x=w161, lower limit=w158) -> (coerced(x)=w159:sgl)  [unwired: 1 out]
            n37 = Subtract(x=w159, y=w158) -> (x-y=w157:sgl)
            n38 = Subtract(x=w160, y=w158) -> (x-y=w156:sgl)
            n39 = Compound Arithmetic op=MULTIPLY(w157, invert w156, sgl 255.0 ("value")) -> (w152:sgl)
            n40 = Index Array(array=w154, index=w152) -> (element=w153:T45)
            n41 = case shown="True" w165 {
              tunnel: w162 -> [w166 w175]
              tunnel: w164 -> [_ w180]
              tunnel: w163 -> [_ w179]
              tunnel: [w168 w183] -> w146
              tunnel: [w167 w182] -> w145
              tunnel: w153 -> [w169 w171]
              tunnel: w151 -> [_ w181]
              tunnel: w150 -> [_ w174]
              tunnel: w149 -> [_ w173]
              tunnel: w148 -> [_ w170]
              tunnel: w144 -> [_ w172]
              frame False {
                n42 = call "IMAQ ColorValueToInteger"("error in (no error)"=w166, "Color Value"=w169) -> ("error out"=w167:errorcluster, "U32 value"=w168:u32)  [unwired: 3 in, 2 out]
              }
              frame True {
                n43 = Index Array(array=w181, index (row)=w180, index (col)=w179) -> (element=w178:sgl)
                n44 = call "Blend Overlay Color with Background.vi"("Overlay Color Value"=w171, "Image Scale Factor"=w170, "Blend Overlay with Background"=w174, "error in (no error)"=w175, "Image Display Range"=w172, "Image Color Array"=w173, "Pixel Value"=w178) -> ("error out"=w176:errorcluster, "Scaled/Blended Overlay Color Value"=w177:T45)  [unwired: 3 in]
                n45 = call "IMAQ ColorValueToInteger"("error in (no error)"=w176, "Color Value"=w177) -> ("error out"=w182:errorcluster, "U32 value"=w183:u32)  [unwired: 3 in, 2 out]
              }
            }
          }
          frame True {
          }
        }
      }
      n46 = Merge Errors(w109) -> (w108:errorcluster)
    }
    n47 = Merge Errors(w60) -> (w58:errorcluster)
    n48 = call "IMAQ Overlay Bitmap"("Group"="Parameter Color Map Overlay", "error in (no error)"=w58, "Bitmap"=w59, "Image"=w61) -> ("error out"=w63:errorcluster, "Image Out"=w105:T3)  [unwired: 6 in]
    n49 = in-place-dvr #1() -> (→"AlliGator IV DVR out":refnum<data-value>, w31:errorcluster)  [unwired: 1 in]
  }
  n50 = call "High Resolution Timing.vi"("relative seconds (NaN)"=w7, "Error In"=w31) -> ("relative seconds"=w5:dbl, "elapsed (relative) seconds"=→"Overlay Compute (s)":dbl, "Error Out"=w8:errorcluster)  [unwired: 15 in]
  n51 = Merge Errors(w8, w3) -> (w4:errorcluster)
  n52 = call "IMAQ Clear Overlay"("error in (no error)"=w4, "Image"=w44) -> ("error out"=w41:errorcluster, "Image Out"=w48:T3)  [unwired: 8 in]
  n53 = Add Array Elements(numeric array=w49) -> (sum=→"# Overlay Pixels":i32)
  n54 = call <vilib>:"Clear Errors.vi"("error in (no error)"=w41, "specific error code to clear (0: all)"=w40) -> ("error out"=w38:errorcluster)  [unwired: 4 in, 1 out]
  n55 = call "High Resolution Timing.vi"("relative seconds (NaN)"=w5, "Error In"=w38) -> ("relative seconds"=w35:dbl, "elapsed (relative) seconds"=→"Overlay Erase (s)":dbl, "Error Out"=w33:errorcluster)  [unwired: 15 in]
  n56 = call "IMAQ Copy Overlay"("error in (no error)"=w33, "Image Dst"=w48, "Image Src"=w30) -> ("error out"=w36:errorcluster, "Image Dst Out"=w47:T3)  [unwired: 7 in]
  n57 = call "High Resolution Timing.vi"("relative seconds (NaN)"=w35, "Error In"=w36) -> ("elapsed (relative) seconds"=→"Overlay Copy (s)":dbl, "Error Out"=w29:errorcluster)  [unwired: 15 in, 1 out]
  n58 = property class="ImageControl"(reference=w50, error in=w29, "Value"=w47) -> (error out=→"Error Out":errorcluster)  [unwired: 1 out]
  n59 = call "Tiny Clear Error.vi"("Error In"=w29) -> ("no Error Out"=w14:errorcluster)  [unwired: 8 in]
  n60 = call "IMAQ Dispose"("Image"=w30, "error in (no error)"=w14) -> ("error out"=w28:errorcluster)  [unwired: 4 in]
  n61 = call <vilib>:"Clear Errors.vi"("error in (no error)"=w28) -> ()  [unwired: 5 in, 2 out]
